vi "Translator.Translate.Controls.vi"(6 "progressbar":refnum<vi>, 7 "group":string, 8 "error in":errorcluster, 9 "font name":string, 10 "Controls out":T1[](array[typedef]), 11 "Translation file":path=path "D:/PL_0125_Sapphire_Automation_branches/SOFTWARE_v1.1-Translation/settings/Translation-Chinese.ini") -> (0 "error out":errorcluster)   [LabVIEW 2016]
uses:
  Translator.ControlData.ctl
  Translator.ControlTypes.ctl
  <vilib>/Utility/miscctls.llb/LVRowAndColumnTypeDef.ctl
  Translator.File.MatchStrings (Single).vi
  Translator.File.MatchStrings (Array).vi
  <vilib>/Utility/config.llb/NI_LVConfig.lvlib
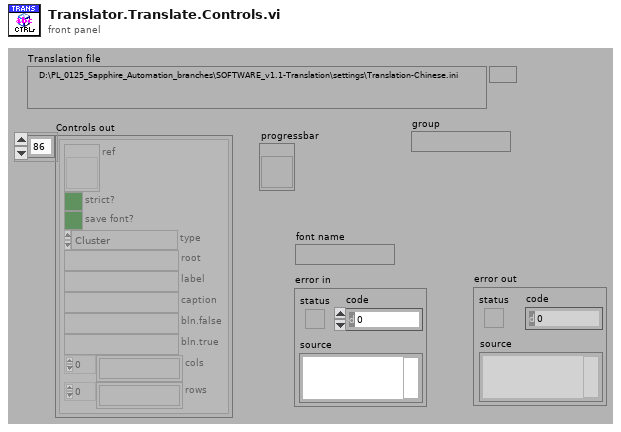
[diagram p1: front panel]
types:
  T1 = typedef "Translator.ControlData.ctl" = cluster{"ref":refnum<vi>, "strict?":bool, "save font?":bool, "type":T2, "root":string, "label":string, "caption":string, "bln.false":string, "bln.true":string, "cols":string[], "rows":string[]}
  T2 = typedef "Translator.ControlTypes.ctl" = enum16{"Cluster", "Array", "Boolean", "Ring", "String", "Tab", "Listbox", "Multicolumn listbox", "Table", "Tree", "Other"}
  T3 = typedef "LVRowAndColumnTypeDef.ctl" = cluster{"Row":i32, "Column":i32}
  T4 = typedef "NI_LVConfig.lvlib/Config Data RefNum.ctl" = refnum<k1>
  T5 = typedef "LVBoundsTypeDef.ctl" = cluster{"Width":u32, "Height":u32}
  T6 = typedef "LVPositionTypeDef.ctl" = cluster{"Left":i32, "Top":i32}
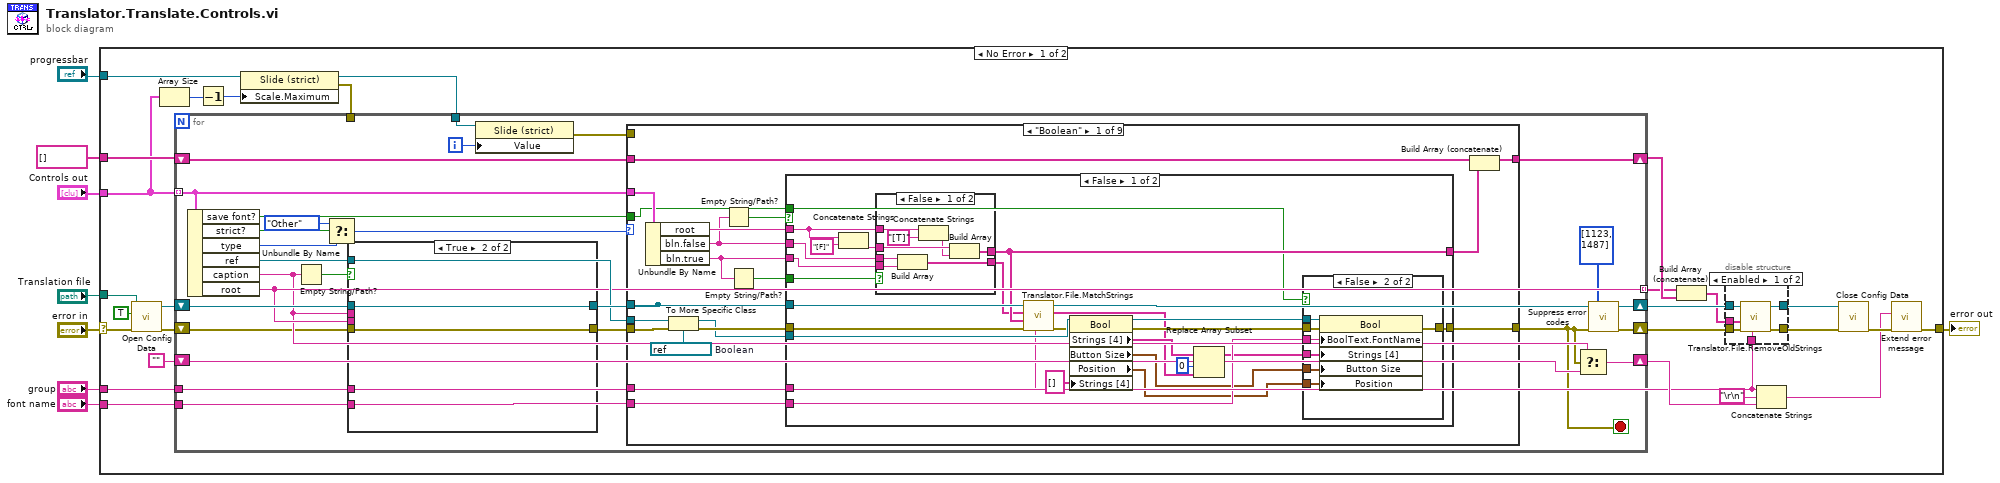
[diagram p0: block diagram]
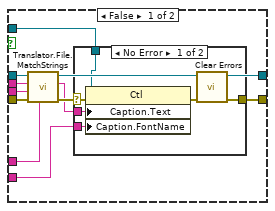
[diagram p3: hidden frame]
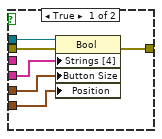
[diagram p5: hidden frame]
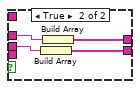
[diagram p6: hidden frame]
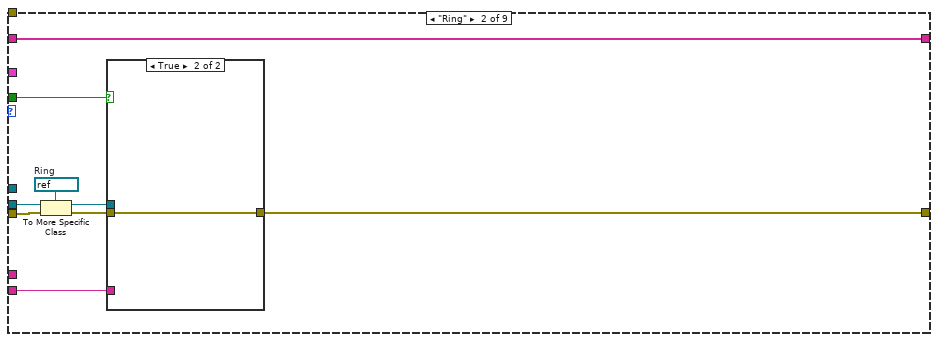
[diagram p8: hidden frame]
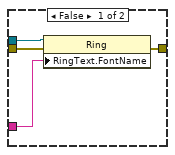
[diagram p9: hidden frame]
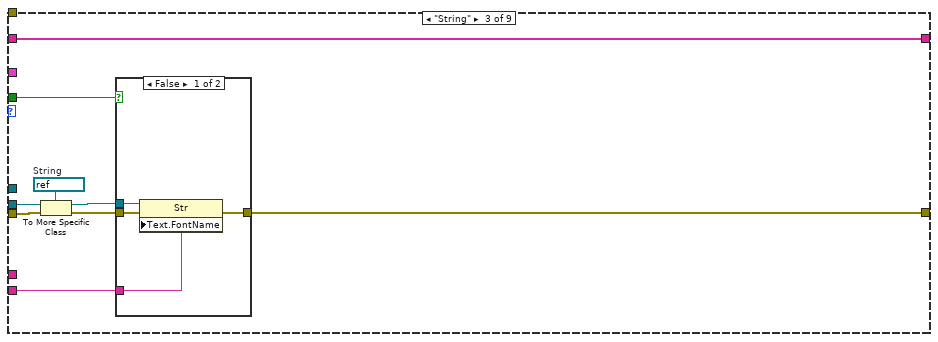
[diagram p10: hidden frame]
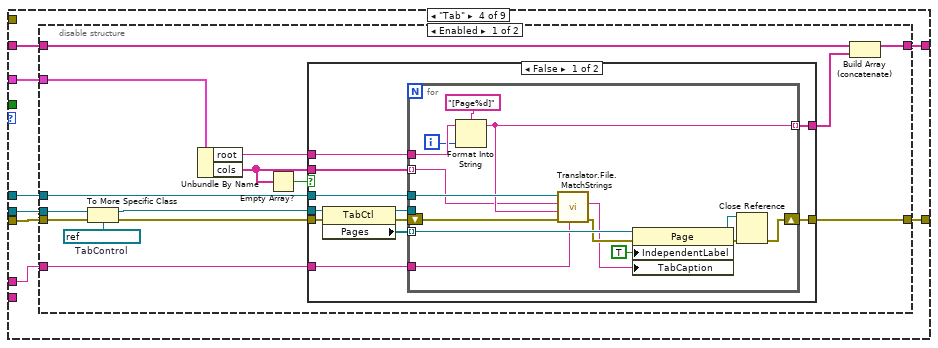
[diagram p12: hidden frame]
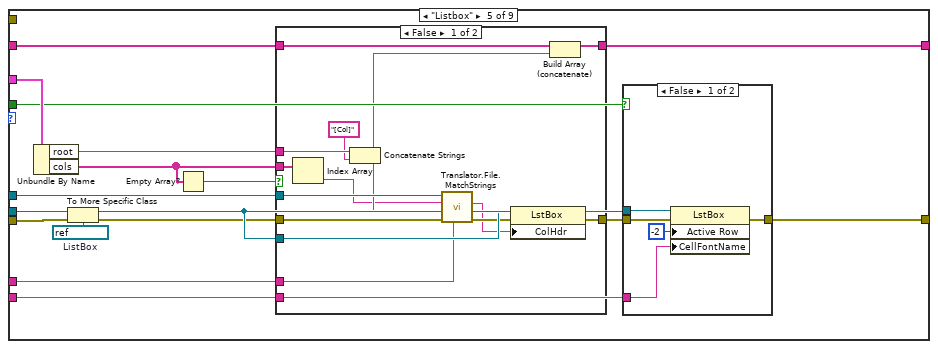
[diagram p15: hidden frame]
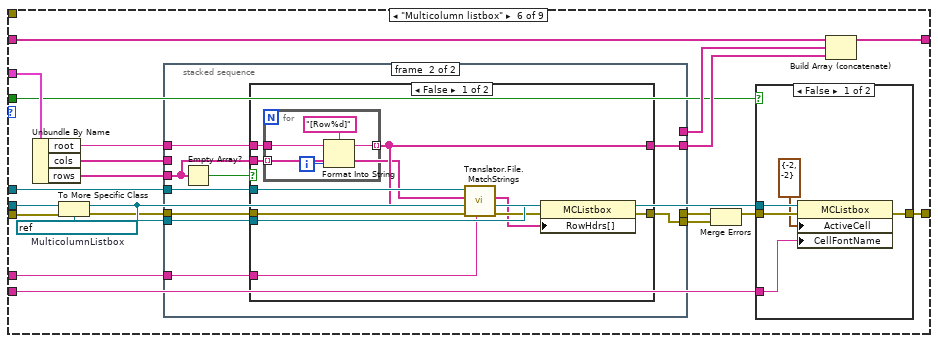
[diagram p18: hidden frame]
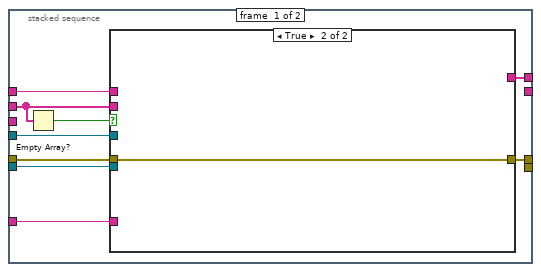
[diagram p20: hidden frame]
diagram:
  n1 = case shown="No Error" "error in" {
    selector: "error in" -> [w19 w506]
    tunnel: "Controls out" -> [w28 _]
    tunnel: [w17 w506] -> w6
    tunnel: "Translation file" -> [w13 _]
    tunnel: "group" -> [w12 _]
    tunnel: "font name" -> [w35 _]
    tunnel: string[] [] -> [w32 _]
    tunnel: "progressbar" -> [w26 _]
    frame No Error {
      n2 = call <vilib>:"Open Config Data.vi"("error in (no error)"=w19, "create file if necessary (T)"=TRUE, "configuration file path"=w13) -> ("error out"=w10:errorcluster, "refnum"=w11:T4)  [unwired: 6 in, 1 out]
      n3 = Array Size(array=w28) -> (size(s)=w27:i32)
      n4 = Decrement(x=w27) -> (x-1=w25:i32)
      n5 = property on="Property Node" class="Slide (strict)"(reference=w26, "Scale.Maximum"=w25) -> (reference out=w24:refnum<vi>, error out=w9:errorcluster)  [unwired: 1 in]
      n6 = for {
        tunnel: w28 -> [w69] mode=indexing
        tunnel: w12 -> [w67]
        shift-right: [w66] -> w34
        shift-left: w11 -> [w68]
        tunnel: w35 -> [w48]
        shift-right: [w57] -> w31
        shift-left: w32 -> [w58]
        tunnel: [w56] -> w30 mode=indexing
        tunnel: w24 -> [w54]
        shift-right: [w51] -> w22
        shift-left: "" -> [w53]
        shift-right: [w50] -> w33
        shift-left: w10 -> [w45]
        tunnel: w9 -> [_]
        i -> [w44]
        stop <- w46 stop-if-true
        n7 = Unbundle By Name(w69) -> ("save font?"=w55:bool, "strict?"=w62:bool, "type"=w61:T2, "ref"=w63:refnum<vi>, "caption"=w52:string, "root"=w56:string)
        n8 = Empty String/Path?(string/path=w52) -> (empty?=w64:bool)
        n9 = Select(t=Translator.ControlTypes."Other", s=w62, f=w61) -> (s? t:f=w59:T2)
        n10 = case shown="True" w64 {
          tunnel: w45 -> [w71 w88]
          tunnel: w68 -> [w79 w87]
          tunnel: w67 -> [w72 _]
          tunnel: [w78 w87] -> w66
          tunnel: [w77 w88] -> w65
          tunnel: w63 -> [w76 _]
          tunnel: w48 -> [w74 _]
          tunnel: w52 -> [w70 _]
          tunnel: w56 -> [w73 _]
          frame False {
            n11 = call-poly "Translator.File.MatchStrings.vi"("group"=w72, "error in"=w71, "label"=w73, "default value"=w70, "refnum in"=w79) -> ("error out"=w77:errorcluster, "value out"=w75:string, "refnum out"=w78:T4)  [unwired: 3 in, 1 out]
            n12 = case shown="No Error" w77 {
              selector: w77 -> [w85 w86]
              tunnel: [w81 w86] -> _
              tunnel: w76 -> [w83 _]
              tunnel: w74 -> [w82 _]
              tunnel: w75 -> [w80 _]
              frame No Error {
                n13 = property class="Ctl"(reference=w83, error in=w85, "Caption.Text"=w80, "Caption.FontName"=w82) -> (error out=w84:errorcluster)  [unwired: 1 out]
                n14 = call <vilib>:"Clear Errors.vi"("error in (no error)"=w84) -> ("error out"=w81:errorcluster)  [unwired: 5 in, 1 out]
              }
              frame Error {
              }
            }
          }
          frame True {
          }
        }
        n15 = property on="Property Node" class="Slide (strict)"(reference=w54, "Value"=w44) -> (error out=w47:errorcluster)  [unwired: 1 in, 1 out]
        n16 = case shown="\"Boolean\"" w59 {
          tunnel: w63 -> [w105 w165 w179 w193 w250 w289 w364 w440 _]
          tunnel: w65 -> [w106 w166 w180 w194 w251 w290 w365 w441 w505]
          tunnel: w69 -> [w104 _ _ w187 w255 w297 w372 w448 _]
          tunnel: [w92 w161 w175 w192 w245 w286 w362 w438 w505] -> w46
          tunnel: w66 -> [w102 _ _ w191 w253 w295 w370 w446 _]
          tunnel: w67 -> [w103 _ _ w190 w252 w293 w368 w444 _]
          tunnel: w48 -> [w91 w162 w176 _ w241 w278 w353 w429 _]
          tunnel: w58 -> [w98 w160 w174 w189 w243 w282 w359 w435 w504]
          tunnel: [w100 w160 w174 w188 w242 w283 w356 w432 w504] -> w57
          tunnel: w55 -> [w89 w159 w173 _ w240 w279 w354 w430 _]
          tunnel: w47 -> [_ _ _ _ _ _ _ _ _]
          frame "Boolean" {
            w107 = refnum<vi> refnum  # Boolean
            n17 = Unbundle By Name(w104) -> ("root"=w101:string, "bln.false"=w97:string, "bln.true"=w96:string)
            n18 = To More Specific Class(target class=w107, reference=w105, error in=w106) -> (specific class reference=w93:refnum<vi>, error out=w94:errorcluster)
            n19 = Empty String/Path?(string/path=w97) -> (empty?=w90:bool)
            n20 = Empty String/Path?(string/path=w96) -> (empty?=w95:bool)
            n21 = case shown="False" w90 {
              tunnel: w93 -> [w126 _]
              tunnel: w94 -> [w111 w158]
              tunnel: [w132 w158] -> w92
              tunnel: w101 -> [w121 _]
              tunnel: w103 -> [w112 _]
              tunnel: w102 -> [w124 _]
              tunnel: [w113 _] -> w99
              tunnel: w96 -> [w119 _]
              tunnel: w97 -> [w120 _]
              tunnel: w95 -> [w123 _]
              tunnel: w91 -> [w118 _]
              tunnel: w89 -> [w108 _]
              frame False {
                n22 = Concatenate Strings(w121, "[F]" ("format string")) -> (w122:string)
                n23 = case shown="False" w123 {
                  tunnel: w121 -> [w152 _]
                  tunnel: [w151 w156] -> w113
                  tunnel: w122 -> [w150 w157]
                  tunnel: w120 -> [w148 w155]
                  tunnel: w119 -> [w147 _]
                  tunnel: [w146 w154] -> w110
                  frame False {
                    n24 = Build Array(w148, w147) -> (w146:string[])
                    n25 = Concatenate Strings(w152, "[T]" ("format string")) -> (w149:string)
                    n26 = Build Array(w150, w149) -> (w151:string[])
                  }
                  frame True {
                    n27 = Build Array(w155) -> (w154:string[])
                    n28 = Build Array(w157) -> (w156:string[])
                  }
                }
                n29 = call-poly "Translator.File.MatchStrings.vi"("group"=w112, "error in"=w111, "labels"=w113, "default values"=w110, "refnum in"=w124) -> ("error out"=w125:errorcluster, "values out"=w115:string[])  [unwired: 3 in, 2 out]
                n30 = property class="Bool"(reference=w126, error in=w125, "Strings [4]"=string[] []) -> (reference out=w128:refnum<vi>, error out=w129:errorcluster, "Strings [4]"=w131:string[], "Button Size"=w116:T5, "Position"=w114:T6)
                n31 = Replace Array Subset(array=w131, new element=w115, index=0) -> (w117:string[])
                n32 = case shown="False" w108 {
                  tunnel: [w138 w145] -> w132
                  tunnel: w129 -> [w137 w144]
                  tunnel: w128 -> [w136 w143]
                  tunnel: w118 -> [_ w142]
                  tunnel: w117 -> [w134 w141]
                  tunnel: w116 -> [w133 w140]
                  tunnel: w114 -> [w135 w139]
                  frame True {
                    n33 = property class="Bool"(reference=w136, error in=w137, "Strings [4]"=w134, "Button Size"=w133, "Position"=w135) -> (error out=w138:errorcluster)  [unwired: 1 out]
                  }
                  frame False {
                    n34 = property class="Bool"(reference=w143, error in=w144, "BoolText.FontName"=w142, "Strings [4]"=w141, "Button Size"=w140, "Position"=w139) -> (error out=w145:errorcluster)  [unwired: 1 out]
                  }
                }
              }
              frame True {
              }
            }
            n35 = Build Array (concatenate)(w98, w99) -> (w100:string[])
          }
          frame "Ring" {
            w167 = refnum<vi> refnum  # Ring
            n36 = To More Specific Class(target class=w167, reference=w165, error in=w166) -> (specific class reference=w164:refnum<vi>, error out=w163:errorcluster)
            n37 = case shown="True" w159 {
              tunnel: w164 -> [w171 _]
              tunnel: w163 -> [w170 w172]
              tunnel: w162 -> [w169 _]
              tunnel: [w168 w172] -> w161
              frame False {
                n38 = property class="Ring"(reference=w171, error in=w170, "RingText.FontName"=w169) -> (error out=w168:errorcluster)  [unwired: 1 out]
              }
              frame True {
              }
            }
          }
          frame "String" {
            w181 = refnum<vi> refnum  # String
            n39 = To More Specific Class(target class=w181, reference=w179, error in=w180) -> (specific class reference=w178:refnum<vi>, error out=w177:errorcluster)
            n40 = case shown="False" w173 {
              tunnel: w178 -> [w185 _]
              tunnel: w177 -> [w184 w186]
              tunnel: w176 -> [w182 _]
              tunnel: [w183 w186] -> w175
              frame False {
                n41 = property class="Str"(reference=w185, error in=w184, "Text.FontName"=w182) -> (error out=w183:errorcluster)  [unwired: 1 out]
              }
              frame True {
              }
            }
          }
          frame "Tab" {
            n42 = disable-structure shown="Enabled" {
              disable-tunnel: w194 -> [w209 w237]
              disable-tunnel: w193 -> [w208 _]
              disable-tunnel: [w207 w237] -> w192
              disable-tunnel: w191 -> [w206 _]
              disable-tunnel: w190 -> [w205 _]
              disable-tunnel: w189 -> [w204 w238]
              disable-tunnel: [w203 w238] -> w188
              disable-tunnel: w187 -> [w195 _]
              frame Enabled {
                w200 = refnum<vi> refnum  # TabControl
                n43 = To More Specific Class(target class=w200, reference=w208, error in=w209) -> (specific class reference=w201:refnum<vi>, error out=w202:errorcluster)
                n44 = Unbundle By Name(w195) -> ("root"=w199:string, "cols"=w198:string[])
                n45 = Empty Array?(array=w198) -> (empty?=w197:bool)
                n46 = case shown="False" w197 {
                  tunnel: w202 -> [w219 w236]
                  tunnel: w201 -> [w216 _]
                  tunnel: [w215 w236] -> w207
                  tunnel: w206 -> [w214 _]
                  tunnel: w199 -> [w213 _]
                  tunnel: w198 -> [w212 _]
                  tunnel: w205 -> [w211 _]
                  tunnel: [w210 _] -> w196
                  frame False {
                    n47 = property class="TabCtl"(reference=w216, error in=w219) -> (reference out=w217:refnum<vi>, error out=w218:errorcluster, "Pages"=w220:refnum<vi>[])
                    n48 = for {
                      tunnel: w220 -> [w235] mode=indexing
                      tunnel: w217 -> [_]
                      shift-right: [w231] -> w215
                      shift-left: w218 -> [w221]
                      tunnel: w212 -> [w222] mode=indexing
                      tunnel: w214 -> [w233]
                      tunnel: w213 -> [w230]
                      tunnel: w211 -> [w224]
                      tunnel: [w223] -> w210 mode=indexing
                      i -> [w228]
                      n49 = Format Into String(format string="[Page%d]", initial string=w230, w228) -> (resulting string=w223:string)  [unwired: 1 in, 1 out]
                      n50 = call-poly "Translator.File.MatchStrings.vi"("group"=w224, "error in"=w221, "label"=w223, "default value"=w222, "refnum in"=w233) -> ("error out"=w234:errorcluster, "value out"=w227:string)  [unwired: 3 in, 2 out]
                      n51 = property class="Page"(reference=w235, error in=w234, "IndependentLabel"=TRUE ("Independent Label"), "TabCaption"=w227) -> (reference out=w226:refnum<vi>, error out=w232:errorcluster)
                      n52 = Close Reference(reference=w226, error in (no error)=w232) -> (error out=w231:errorcluster)
                    }
                  }
                  frame True {
                  }
                }
                n53 = Build Array (concatenate)(w204, w196) -> (w203:string[])
              }
              frame Disabled {
              }
            }
          }
          frame "Listbox" {
            w249 = refnum<vi> refnum  # ListBox
            n54 = Unbundle By Name(w255) -> ("root"=w254:string, "cols"=w248:string[])
            n55 = To More Specific Class(target class=w249, reference=w250, error in=w251) -> (specific class reference=w247:refnum<vi>, error out=w244:errorcluster)
            n56 = Empty Array?(array=w248) -> (empty?=w239:bool)
            n57 = case shown="False" w239 {
              tunnel: [w275 w277] -> w246
              tunnel: w244 -> [w262 w277]
              tunnel: w254 -> [w274 _]
              tunnel: w248 -> [w269 _]
              tunnel: w253 -> [w273 _]
              tunnel: w252 -> [w264 _]
              tunnel: w247 -> [w272 _]
              tunnel: w243 -> [w267 w276]
              tunnel: [w266 w276] -> w242
              tunnel: w241 -> [_ _]
              frame False {
                n58 = Index Array(array=w269) -> (element=w263:string)  [unwired: 1 in]
                n59 = Concatenate Strings(w274, "[Col]" ("format string")) -> (w265:string)
                n60 = call-poly "Translator.File.MatchStrings.vi"("group"=w264, "error in"=w262, "label"=w265, "default value"=w263, "refnum in"=w273) -> ("error out"=w271:errorcluster, "value out"=w268:string)  [unwired: 3 in, 2 out]
                n61 = property class="LstBox"(reference=w272, error in=w271, "ColHdr"=w268) -> (error out=w275:errorcluster)  [unwired: 1 out]
                n62 = Build Array (concatenate)(w267, w265) -> (w266:string[])
              }
              frame True {
              }
            }
            n63 = case shown="False" w240 {
              tunnel: w247 -> [w260 _]
              tunnel: w246 -> [w259 w261]
              tunnel: w241 -> [w257 _]
              tunnel: [w256 w261] -> w245
              frame False {
                n64 = property class="LstBox"(reference=w260, error in=w259, "Active Row"=-2 ("Active Row:Active Row Number"), "CellFontName"=w257) -> (error out=w256:errorcluster)  [unwired: 1 out]
              }
              frame True {
              }
            }
          }
          frame "Multicolumn listbox" {
            w288 = refnum<vi> refnum  # MulticolumnListbox
            n65 = Unbundle By Name(w297) -> ("root"=w296:string, "cols"=w294:string[], "rows"=w292:string[])
            n66 = To More Specific Class(target class=w288, reference=w289, error in=w290) -> (specific class reference=w285:refnum<vi>, error out=w284:errorcluster)
            n67 = stacked-sequence {
              tunnel: [w307 _] -> w298
              tunnel: w284 -> [w313 w337]
              tunnel: w296 -> [w312 w336]
              tunnel: w295 -> [w311 w335]
              tunnel: w294 -> [w308 _]
              tunnel: w293 -> [w310 w334]
              tunnel: w292 -> [_ w333]
              tunnel: [_ w330] -> w291
              tunnel: w285 -> [w309 w332]
              tunnel: [w306 _] -> w281
              tunnel: [_ w331] -> w280
              frame #0 {
                n68 = Empty Array?(array=w308) -> (empty?=w305:bool)
                n69 = case shown="True" w305 {
                  tunnel: [w323 w328] -> w307
                  tunnel: w313 -> [w315 w328]
                  tunnel: w312 -> [w322 _]
                  tunnel: w308 -> [w314 _]
                  tunnel: w311 -> [w321 _]
                  tunnel: w310 -> [w317 _]
                  tunnel: w309 -> [w320 _]
                  tunnel: [w316 _] -> w306
                  frame False {
                    n70 = for {
                      tunnel: w322 -> [w326]
                      tunnel: [w324] -> w316 mode=indexing
                      tunnel: w314 -> [_] mode=indexing
                      i -> [w325]
                      n71 = Format Into String(format string="[Col%d]", initial string=w326, w325) -> (resulting string=w324:string)  [unwired: 1 in, 1 out]
                    }
                    n72 = call-poly "Translator.File.MatchStrings.vi"("group"=w317, "error in"=w315, "labels"=w316, "default values"=w314, "refnum in"=w321) -> ("error out"=w319:errorcluster, "values out"=w318:string[])  [unwired: 3 in, 2 out]
                    n73 = property class="MCListbox"(reference=w320, error in=w319, "ColHdrString"=w318) -> (error out=w323:errorcluster)  [unwired: 1 out]
                  }
                  frame True {
                  }
                }
              }
              frame #1 {
                n74 = Empty Array?(array=w333) -> (empty?=w329:bool)
                n75 = case shown="False" w329 {
                  tunnel: [w347 w352] -> w330
                  tunnel: w337 -> [w338 w352]
                  tunnel: w336 -> [w346 _]
                  tunnel: w333 -> [w339 _]
                  tunnel: w335 -> [w345 _]
                  tunnel: w334 -> [w341 _]
                  tunnel: w332 -> [w344 _]
                  tunnel: [w340 _] -> w331
                  frame False {
                    n76 = for {
                      tunnel: w346 -> [w350]
                      tunnel: [w348] -> w340 mode=indexing
                      tunnel: w339 -> [_] mode=indexing
                      i -> [w349]
                      n77 = Format Into String(format string="[Row%d]", initial string=w350, w349) -> (resulting string=w348:string)  [unwired: 1 in, 1 out]
                    }
                    n78 = call-poly "Translator.File.MatchStrings.vi"("group"=w341, "error in"=w338, "labels"=w340, "default values"=w339, "refnum in"=w345) -> ("error out"=w343:errorcluster, "values out"=w342:string[])  [unwired: 3 in, 2 out]
                    n79 = property class="MCListbox"(reference=w344, error in=w343, "RowHdrs[]"=w342) -> (error out=w347:errorcluster)  [unwired: 1 out]
                  }
                  frame True {
                  }
                }
              }
            }
            n80 = Merge Errors(w298, w291) -> (w287:errorcluster)
            n81 = case shown="False" w279 {
              tunnel: w287 -> [w303 w304]
              tunnel: [w302 w304] -> w286
              tunnel: w285 -> [w301 _]
              tunnel: w278 -> [w299 _]
              frame False {
                n82 = property class="MCListbox"(reference=w301, error in=w303, "ActiveCell"=T3 {"Row"=-2, "Column"=-2} ("Active Cell:Active Cell"), "CellFontName"=w299) -> (error out=w302:errorcluster)  [unwired: 1 out]
              }
              frame True {
              }
            }
            n83 = Build Array (concatenate)(w282, w281, w280) -> (w283:string[])
          }
          frame "Table" {
            w361 = refnum<vi> refnum  # Table
            n84 = Unbundle By Name(w372) -> ("root"=w371:string, "cols"=w369:string[], "rows"=w367:string[])
            n85 = To More Specific Class(target class=w361, reference=w364, error in=w365) -> (specific class reference=w355:refnum<vi>, error out=w360:errorcluster)
            n86 = stacked-sequence {
              tunnel: [w382 _] -> w373
              tunnel: w360 -> [w388 w412]
              tunnel: w371 -> [w387 w411]
              tunnel: w370 -> [w386 w410]
              tunnel: w369 -> [w383 _]
              tunnel: w368 -> [w385 w409]
              tunnel: w367 -> [_ w408]
              tunnel: [_ w406] -> w366
              tunnel: w355 -> [w384 w407]
              tunnel: [_ w405] -> w358
              tunnel: [w381 _] -> w357
              frame #0 {
                n87 = Empty Array?(array=w383) -> (empty?=w380:bool)
                n88 = case shown="False" w380 {
                  tunnel: [w398 w403] -> w382
                  tunnel: w388 -> [w389 w403]
                  tunnel: w387 -> [w397 _]
                  tunnel: w383 -> [w390 _]
                  tunnel: w386 -> [w396 _]
                  tunnel: w385 -> [w392 _]
                  tunnel: w384 -> [w395 _]
                  tunnel: [w391 _] -> w381
                  frame False {
                    n89 = for {
                      tunnel: w397 -> [w401]
                      tunnel: [w399] -> w391 mode=indexing
                      tunnel: w390 -> [_] mode=indexing
                      i -> [w400]
                      n90 = Format Into String(format string="[Col%d]", initial string=w401, w400) -> (resulting string=w399:string)  [unwired: 1 in, 1 out]
                    }
                    n91 = call-poly "Translator.File.MatchStrings.vi"("group"=w392, "error in"=w389, "labels"=w391, "default values"=w390, "refnum in"=w396) -> ("error out"=w394:errorcluster, "values out"=w393:string[])  [unwired: 3 in, 2 out]
                    n92 = property class="Tbl"(reference=w395, error in=w394, "Column Headers[]"=w393) -> (error out=w398:errorcluster)  [unwired: 1 out]
                  }
                  frame True {
                  }
                }
              }
              frame #1 {
                n93 = Empty Array?(array=w408) -> (empty?=w404:bool)
                n94 = case shown="False" w404 {
                  tunnel: [w423 w428] -> w406
                  tunnel: w412 -> [w414 w428]
                  tunnel: w411 -> [w422 _]
                  tunnel: w408 -> [w413 _]
                  tunnel: w410 -> [w421 _]
                  tunnel: w409 -> [w416 _]
                  tunnel: w407 -> [w420 _]
                  tunnel: [w417 _] -> w405
                  frame False {
                    n95 = for {
                      tunnel: w422 -> [w426]
                      tunnel: [w424] -> w417 mode=indexing
                      tunnel: w413 -> [_] mode=indexing
                      tunnel: [w424] -> w415 mode=indexing
                      i -> [w425]
                      n96 = Format Into String(format string="[Row%d]", initial string=w426, w425) -> (resulting string=w424:string)  [unwired: 1 in, 1 out]
                    }
                    n97 = call-poly "Translator.File.MatchStrings.vi"("group"=w416, "error in"=w414, "labels"=w415, "default values"=w413, "refnum in"=w421) -> ("error out"=w419:errorcluster, "values out"=w418:string[])  [unwired: 3 in, 2 out]
                    n98 = property class="Tbl"(reference=w420, error in=w419, "Row Headers[]"=w418) -> (error out=w423:errorcluster)  [unwired: 1 out]
                  }
                  frame True {
                  }
                }
              }
            }
            n99 = Merge Errors(w373, w366) -> (w363:errorcluster)
            n100 = case shown="False" w354 {
              tunnel: w363 -> [w378 w379]
              tunnel: [w377 w379] -> w362
              tunnel: w353 -> [w375 _]
              tunnel: w355 -> [w374 _]
              frame False {
                n101 = property class="Tbl"(reference=w374, error in=w378, "Active Cell"=T3 {"Row"=-2, "Column"=-2} ("Active Cell:Active Cell"), "CellFontName"=w375) -> (error out=w377:errorcluster)  [unwired: 1 out]
              }
              frame True {
              }
            }
            n102 = Build Array (concatenate)(w359, w357, w358) -> (w356:string[])
          }
          frame "Tree" {
            w437 = refnum<vi> refnum  # TreeControl
            n103 = Unbundle By Name(w448) -> ("root"=w447:string, "cols"=w445:string[], "rows"=w443:string[])
            n104 = To More Specific Class(target class=w437, reference=w440, error in=w441) -> (specific class reference=w431:refnum<vi>, error out=w436:errorcluster)
            n105 = stacked-sequence {
              tunnel: [w458 _] -> w449
              tunnel: w436 -> [w464 w488]
              tunnel: w447 -> [w463 w487]
              tunnel: w446 -> [w462 w486]
              tunnel: w445 -> [w459 _]
              tunnel: w444 -> [w461 w485]
              tunnel: w443 -> [_ w484]
              tunnel: [_ w482] -> w442
              tunnel: w431 -> [w460 w483]
              tunnel: [_ w481] -> w434
              tunnel: [w457 _] -> w433
              frame #0 {
                n106 = Empty Array?(array=w459) -> (empty?=w456:bool)
                n107 = case shown="False" w456 {
                  tunnel: [w474 w479] -> w458
                  tunnel: w464 -> [w465 w479]
                  tunnel: w463 -> [w473 _]
                  tunnel: w459 -> [w466 _]
                  tunnel: w462 -> [w472 _]
                  tunnel: w461 -> [w468 _]
                  tunnel: w460 -> [w471 _]
                  tunnel: [w467 _] -> w457
                  frame False {
                    n108 = for {
                      tunnel: w473 -> [w477]
                      tunnel: [w475] -> w467 mode=indexing
                      tunnel: w466 -> [_] mode=indexing
                      i -> [w476]
                      n109 = Format Into String(format string="[Col%d]", initial string=w477, w476) -> (resulting string=w475:string)  [unwired: 1 in, 1 out]
                    }
                    n110 = call-poly "Translator.File.MatchStrings.vi"("group"=w468, "error in"=w465, "labels"=w467, "default values"=w466, "refnum in"=w472) -> ("error out"=w470:errorcluster, "values out"=w469:string[])  [unwired: 3 in, 2 out]
                    n111 = property class="Tree"(reference=w471, error in=w470, "ColHdrString"=w469) -> (error out=w474:errorcluster)  [unwired: 1 out]
                  }
                  frame True {
                  }
                }
              }
              frame #1 {
                n112 = Empty Array?(array=w484) -> (empty?=w480:bool)
                n113 = case shown="False" w480 {
                  tunnel: [w498 w503] -> w482
                  tunnel: w488 -> [w490 w503]
                  tunnel: w487 -> [w497 _]
                  tunnel: w484 -> [w489 _]
                  tunnel: w486 -> [w496 _]
                  tunnel: w485 -> [w492 _]
                  tunnel: w483 -> [w495 _]
                  tunnel: [w491 _] -> w481
                  frame False {
                    n114 = for {
                      tunnel: w497 -> [w501]
                      tunnel: w489 -> [_] mode=indexing
                      tunnel: [w499] -> w491 mode=indexing
                      i -> [w500]
                      n115 = Format Into String(format string="[Row%d]", initial string=w501, w500) -> (resulting string=w499:string)  [unwired: 1 in, 1 out]
                    }
                    n116 = call-poly "Translator.File.MatchStrings.vi"("group"=w492, "error in"=w490, "labels"=w491, "default values"=w489, "refnum in"=w496) -> ("error out"=w494:errorcluster, "values out"=w493:string[])  [unwired: 3 in, 2 out]
                    n117 = property class="Tree"(reference=w495, error in=w494, "RowHdrs[]"=w493) -> (error out=w498:errorcluster)  [unwired: 1 out]
                  }
                  frame True {
                  }
                }
              }
            }
            n118 = Merge Errors(w449, w442) -> (w439:errorcluster)
            n119 = case shown="False" w430 {
              tunnel: w439 -> [w454 w455]
              tunnel: [w453 w455] -> w438
              tunnel: w429 -> [w451 _]
              tunnel: w431 -> [w452 _]
              frame False {
                w450 = -2 ("Active Cell:Active Column Number")
                n120 = property class="Tree"(reference=w452, error in=w454, "Active Item Row Number"=w450, "ActiveColNum"=w450, "CellFontName"=w451) -> (error out=w453:errorcluster)  [unwired: 1 out]
              }
              frame True {
              }
            }
            n121 = Build Array (concatenate)(w435, w433, w434) -> (w432:string[])
          }
          frame Default {
          }
        }
        n122 = Select(t=w52, s=w46, f=w53) -> (s? t:f=w51:string)
        n123 = call "Suppress error codes.vi"("error in (no error)"=w46, "suppress codes([43])"=i32[] [1123, 1487]) -> ("error out"=w50:errorcluster)  [unwired: 8 in, 1 out]
      }
      n124 = Build Array (concatenate)(w30, w31) -> (w29:string[])
      n125 = disable-structure shown="Enabled" {
        disable-tunnel: w34 -> [w41 w43]
        disable-tunnel: w33 -> [w40 w42]
        disable-tunnel: [w39 w42] -> w14
        disable-tunnel: w29 -> [w38 _]
        disable-tunnel: [w37 w43] -> w16
        disable-tunnel: w12 -> [w36 _]
        frame Enabled {
          n126 = call "Translator.File.RemoveOldStrings.vi"("group"=w36, "error in"=w40, "labels"=w38, "refnum in"=w41) -> ("error out"=w39:errorcluster, "refnum out"=w37:T4)  [unwired: 5 in, 1 out]
        }
        frame Disabled {
        }
      }
      n127 = Concatenate Strings(w12, "\r\n", w22) -> (w15:string)
      n128 = call <vilib>:"Close Config Data.vi"("error in (no error)"=w14, "refnum"=w16) -> ("error out"=w18:errorcluster)  [unwired: 8 in, 1 out]
      n129 = call "Extend error message.vi"("error in"=w18, "extra message part"=w15) -> ("error out"=w17:errorcluster)  [unwired: 9 in]
    }
    frame Error {
    }
  }
  "error out" <- w6
